vi "success.vi"() -> ()   [LabVIEW 2024]
uses:
  <vilib>/Instr/_visa.llb/VISA Configure Serial Port (Instr).vi
  <vilib>/addons/control/pid/pid.llb/PID (DBL).vi
  <vilib>/addons/control/pid/NI_PID_pid.lvlib
panel:
  out "LEVEL":dbl
  out "Waveform Chart":dbl(graph)
  out "error":dbl
  in  "Set point":i32
  out "output":dbl
  in  "stop":bool
  in  "VISA resource name":refnum<visa-resource-name>="COM7"
  out "DISTANCE":string
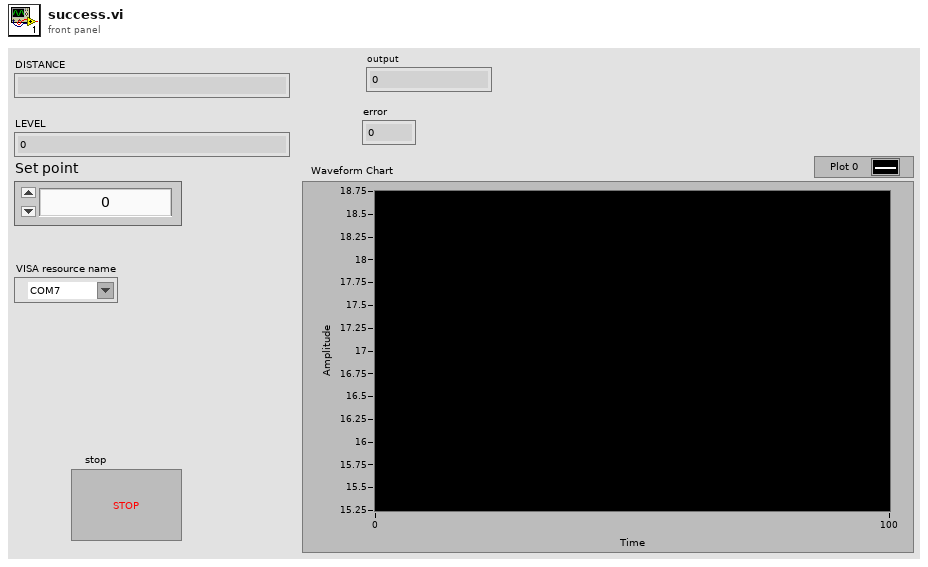
[diagram p1: front panel]
types:
  T1 = cluster{"proportional gain (Kc)":dbl, "integral time (Ti, min)":dbl, "derivative time (Td, min)":dbl}
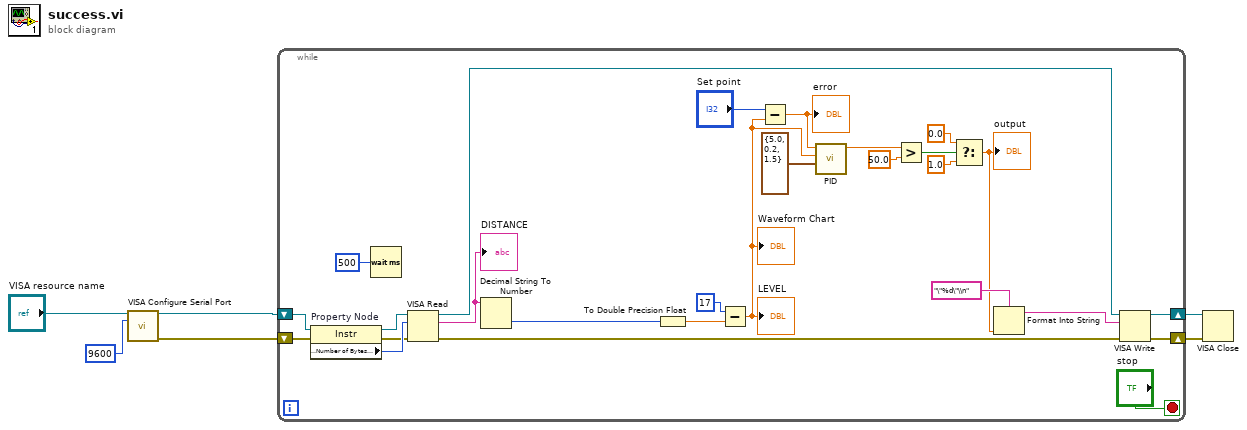
[diagram p0: block diagram]
diagram:
  n1 = call-poly "VISA Configure Serial Port"("VISA resource name"="VISA resource name", "baud rate (9600)"=u32 9600) -> ("VISA resource name out"=w6:refnum<visa-resource-name>, "error out"=w5:errorcluster)  [unwired: 12 in]
  n2 = while {
    shift-right: [w18] -> w4
    shift-left: w6 -> [w33]
    shift-right: [w17] -> w3
    shift-left: w5 -> [w30]
    stop <- "stop" stop-if-true
    n3 = property on="Property Node" class="Instr"(reference=w33, error in=w30) -> (reference out=w32:refnum<visa-resource-name>, error out=w29:errorcluster, "Serial Settings:Number of Bytes at Serial Port"=w31:u32)
    n4 = Wait (ms)(milliseconds to wait=u32 500) -> ()  [unwired: 1 out]
    n5 = VISA Read(VISA resource name=w32, byte count=w31, error in (no error)=w29) -> (VISA resource name out=w16:refnum<visa-resource-name>, read buffer=w19:string, error out=w15:errorcluster)  [unwired: 1 out]
    "DISTANCE" <- w19
    n6 = Decimal String To Number(string=w19) -> (number=w22:i32)  [unwired: 2 in, 1 out]
    n7 = To Double Precision Float(number=w22) -> (double precision float=w21:dbl)
    n8 = Subtract(x=17 ("y"), y=w21) -> (x-y=w8:dbl)
    "Waveform Chart" <- w8
    "LEVEL" <- w8
    n9 = Subtract(x="Set point", y=w8) -> (x-y=w13:dbl)
    "error" <- w13
    n10 = call-poly <vilib>:"PID.vi"("PID gains"=T1 {"proportional gain (Kc)"=5.0, "integral time (Ti, min)"=0.2, "derivative time (Td, min)"=1.5}, "process variable"=w8, "setpoint"=w13) -> ("output"=w14:dbl)  [unwired: 7 in, 1 out]
    n11 = Greater?(x=w14, y=50.0) -> (0:w9:bool)
    n12 = Select(t=0.0, s=w9, f=1.0) -> (s? t:f=w23:dbl)
    "output" <- w23
    n13 = Format Into String "Format Into String"(format string="\"%d\"\\n" ("initial string"), w23) -> (resulting string=w27:string)  [unwired: 2 in, 1 out]
    n14 = VISA Write(VISA resource name=w16, write buffer=w27, error in (no error)=w15) -> (VISA resource name out=w18:refnum<visa-resource-name>, error out=w17:errorcluster)  [unwired: 1 out]
  }
  n15 = VISA Close(VISA resource name=w4, error in (no error)=w3) -> ()  [unwired: 1 out]
